vi "blue.vi"() -> (3 "blue 5":i32)   [LabVIEW 2019]
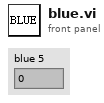
[diagram p1: front panel]
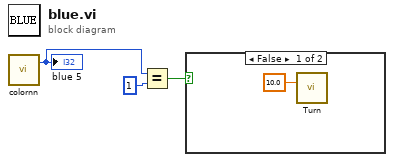
[diagram p0: block diagram]
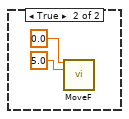
[diagram p2: hidden frame]
diagram:
  n1 = call "colornn.vi"() -> ("blue"=w3:i32)  [unwired: 14 in, 5 out]
  "blue 5" <- w3
  n2 = Equal?(x=w3, y=1) -> (x = y?=w2:bool)
  n3 = case shown="False" w2 {
    frame False {
      n4 = call "Turn.vi"("¨¤«×"=10.0) -> ()  [unwired: 14 in, 1 out]
    }
    frame True {
      n5 = call "MoveF.vi"("X"=0.0, "Y"=5.0) -> ()  [unwired: 13 in, 1 out]
    }
  }
